vi "Main_System.back.vi"(7 "LabVIEW Web Service Request":refnum<class "Web Request.lvclass">) -> ()   [LabVIEW 2016]
uses:
  <vilib>/wsapi/Web Request.lvclass
  SubVIs/System_States.ctl
panel:
  in  "Tab Control":enum32{"Page 1", "Page 2"}(tab)
  out "error IO":errorcluster
  out "JSON string":string
  out "runtime":dbl=-1.0 format="%#_13g"
  out "Cluster":T1
  in  "Debug Provide Metadata":bool
  in  "Debug Provide Metadata (file)":bool
  out "Next State":T2
  out "Output/Debug":T3={"Test_File"="", "Error"="OK", "RF_Center_Freq"="0", "RF_Gain"="0", "Status"="Done"}
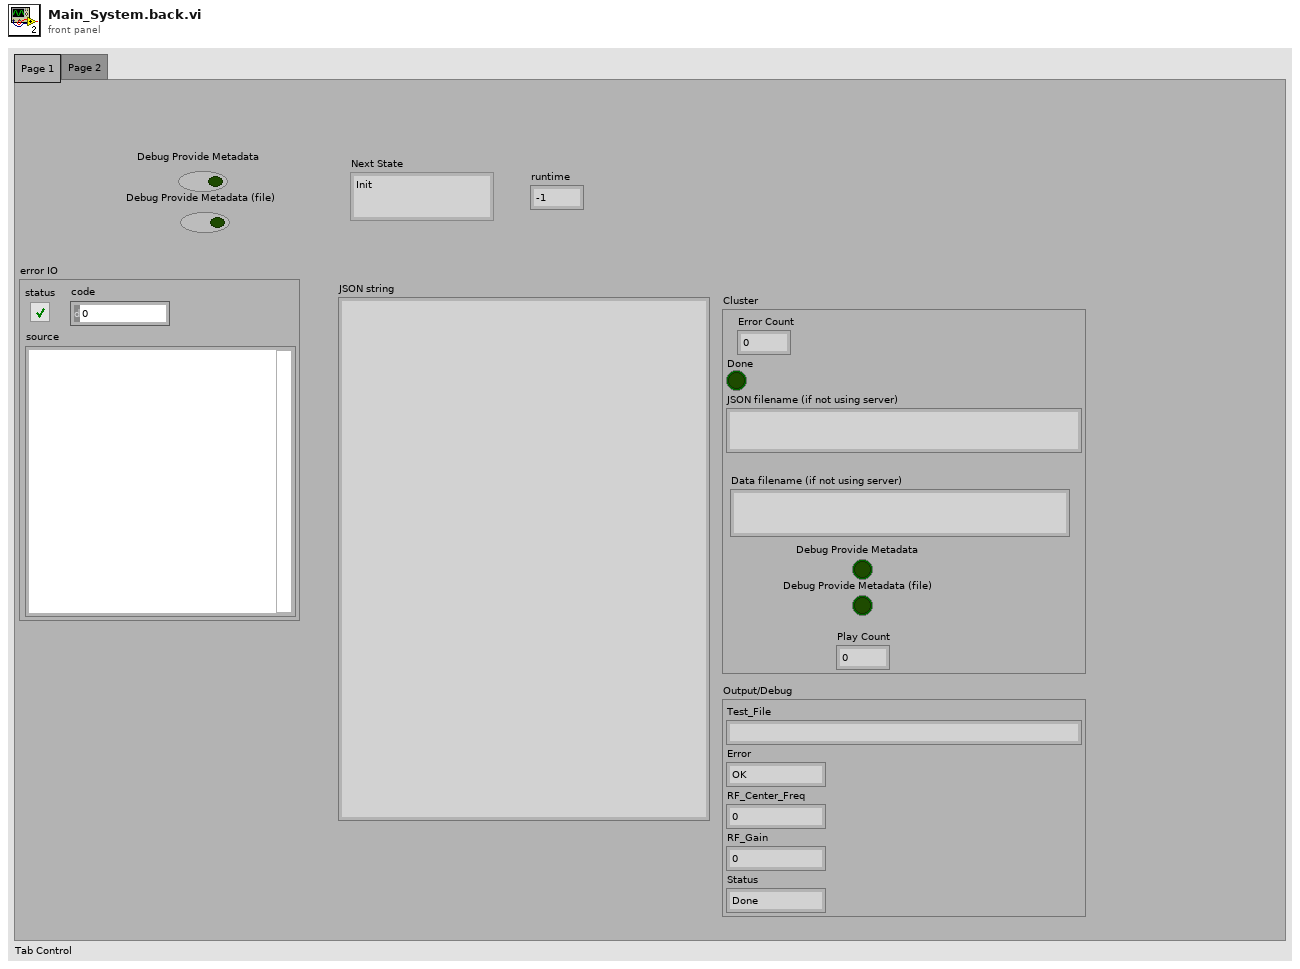
[diagram p1: front panel]
types:
  T1 = cluster{"Error Count":u64, "Done":bool, "JSON filename (if not using server)":string, "Data filename (if not using server)":string, "Debug Provide Metadata":bool, "Debug Provide Metadata (file)":bool, "Play Count":u64}
  T2 = typedef "System_States.ctl" = enum16{"Init", "Wait for Metadata", "Parse Metadata", "Play File", "Finished Playing", "Report Error", "Exit"}
  T3 = cluster{"Test_File":string, "Error":string, "RF_Center_Freq":string, "RF_Gain":string, "Status":string}
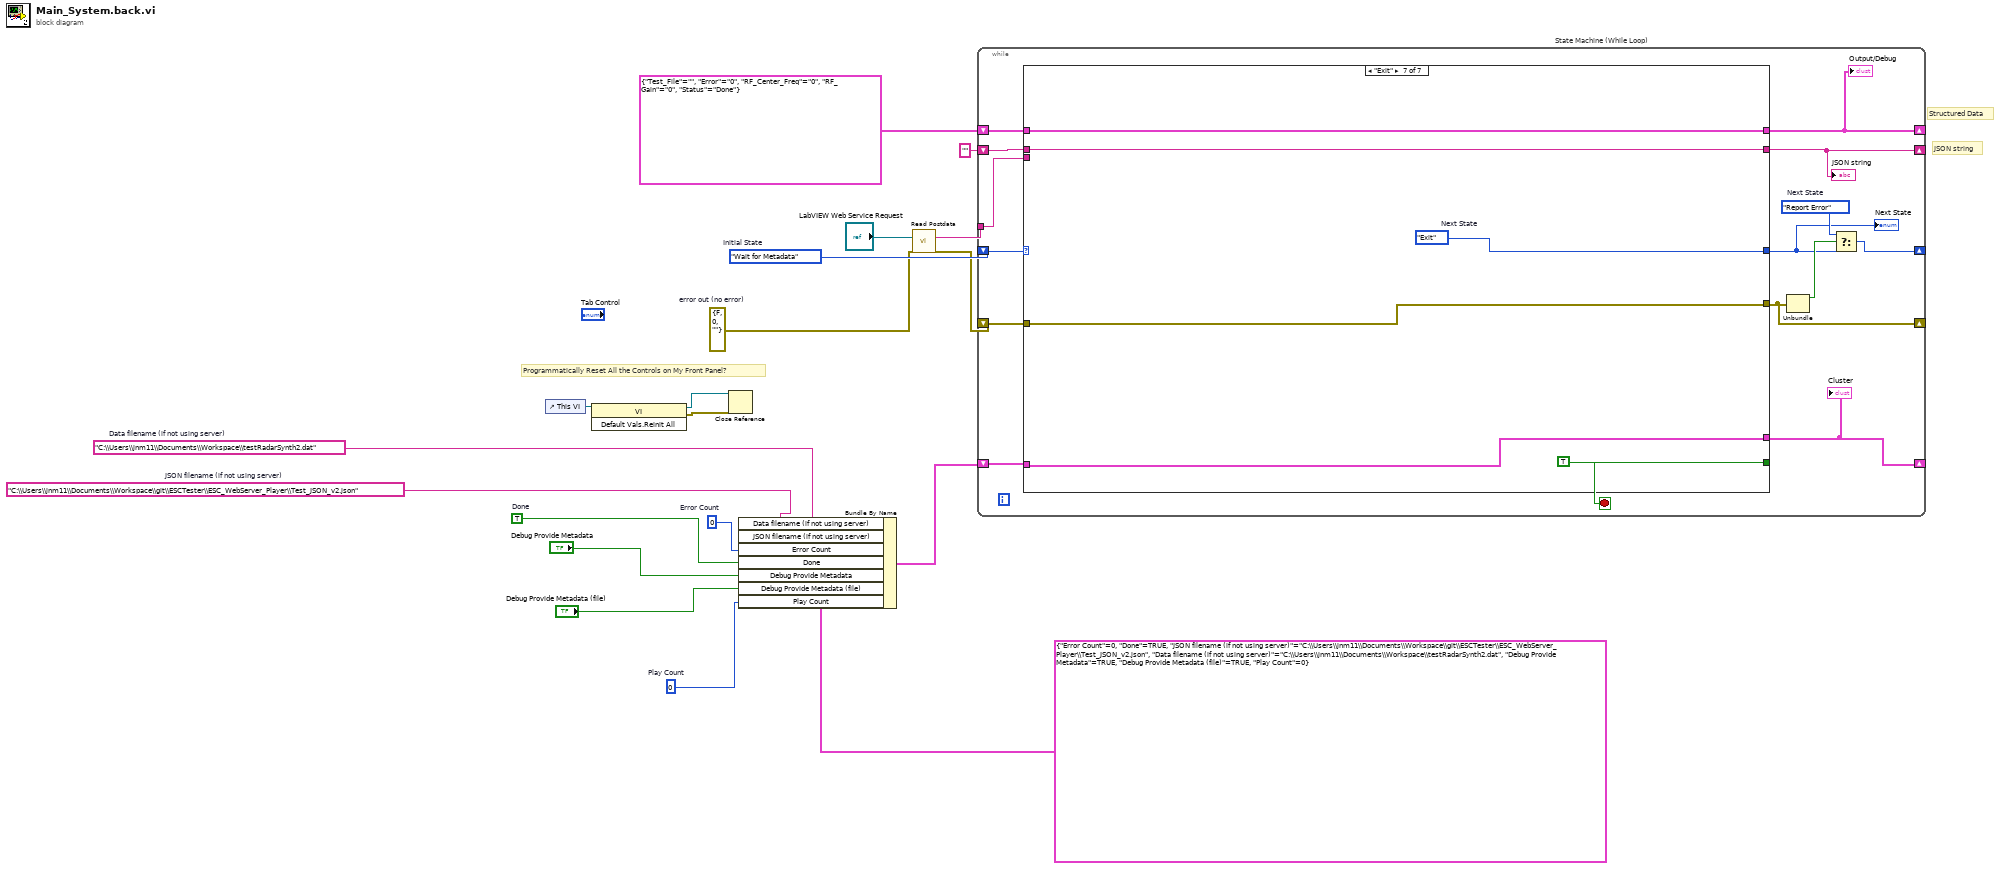
[diagram p0: block diagram]
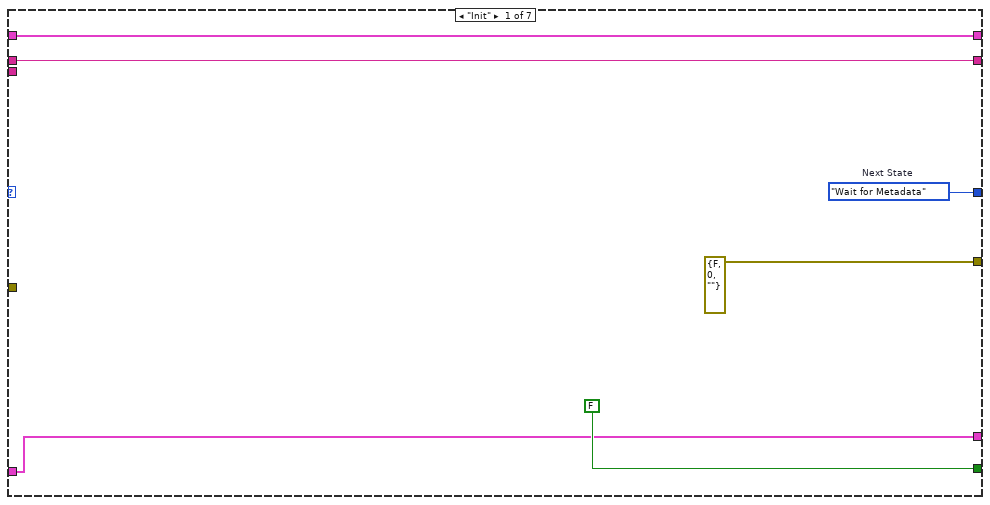
[diagram p2: hidden frame]
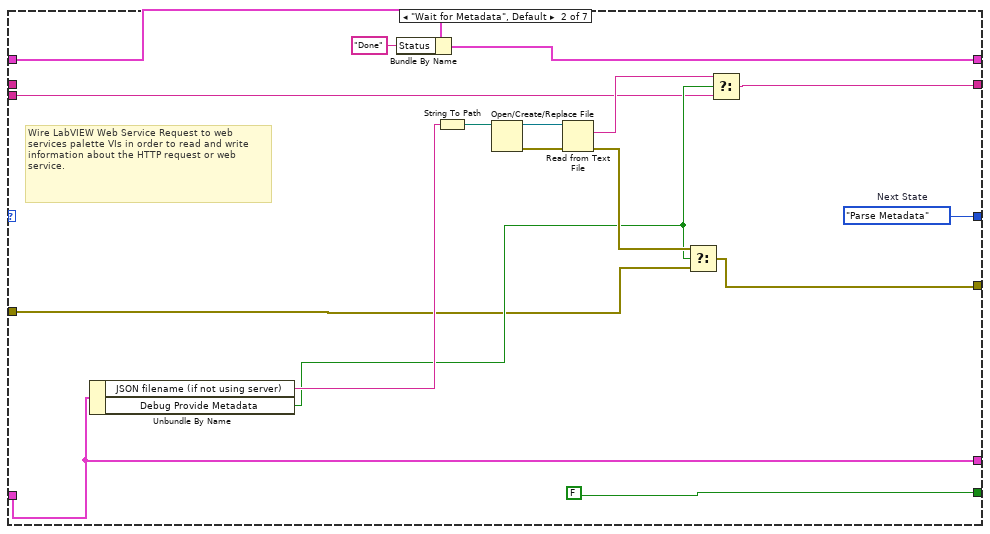
[diagram p3: hidden frame]
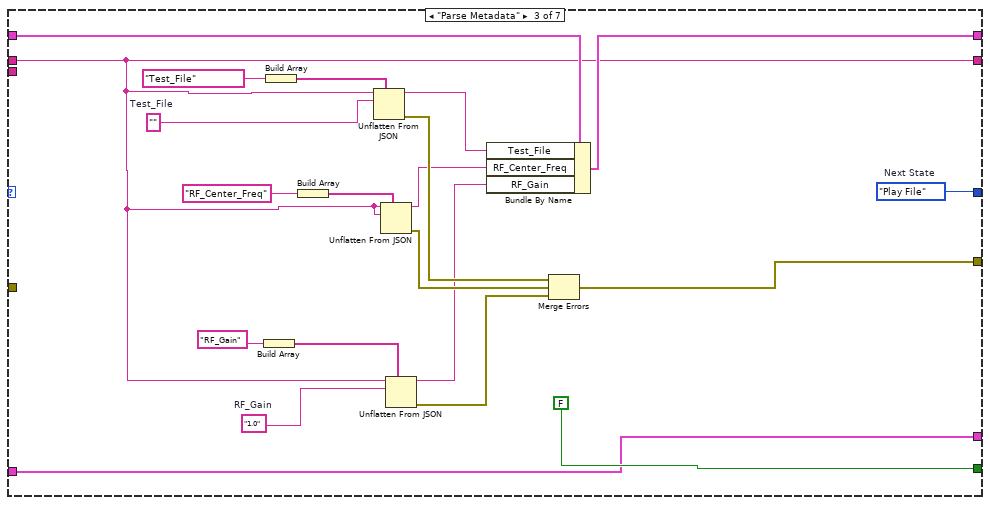
[diagram p4: hidden frame]
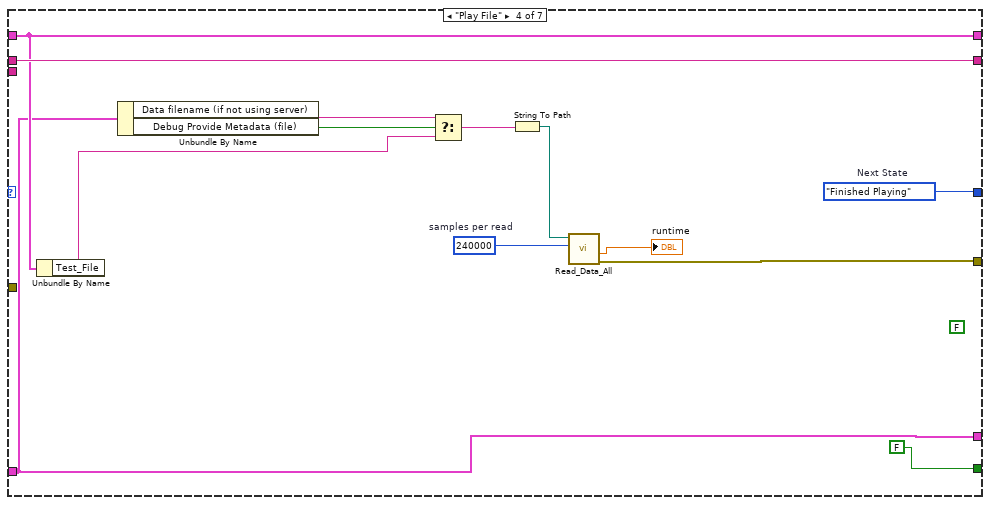
[diagram p5: hidden frame]
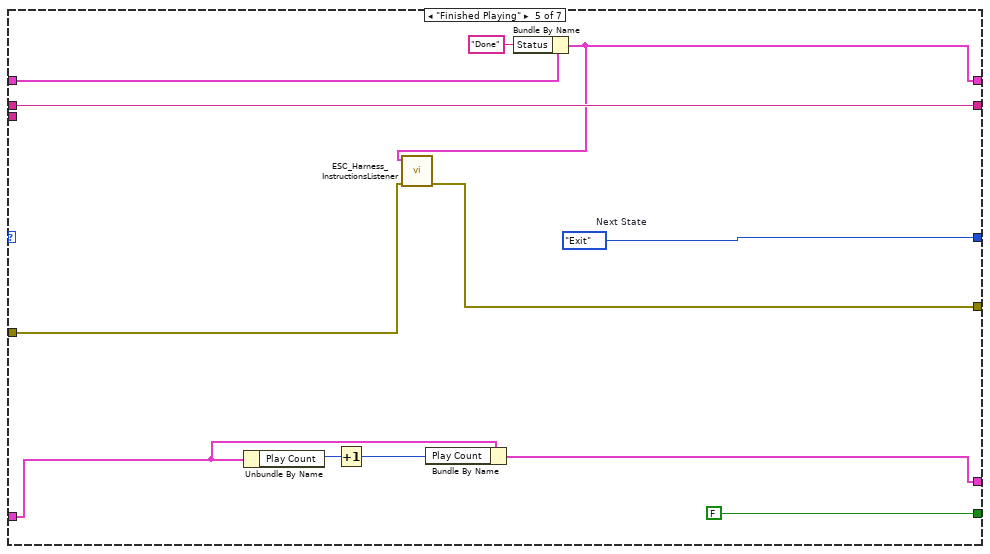
[diagram p6: hidden frame]
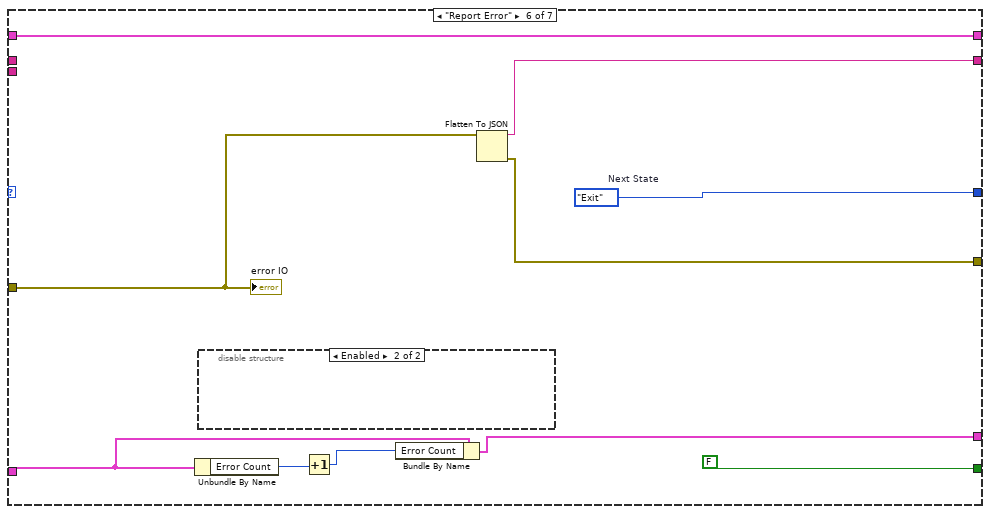
[diagram p7: hidden frame]
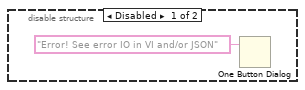
[diagram p8: hidden frame]
diagram:
  w9 = u64 0  # Play Count
  w15 = TRUE  # Done
  w16 = u64 0  # Error Count
  w10 = "C:\\Users\\jnm11\\Documents\\Workspace\\testRadarSynth2.dat"  # Data filename (if not using server)
  w17 = "C:\\Users\\jnm11\\Documents\\Workspace\\git\\ESCTester\\ESC_WebServer_Player\\Test_JSON_v2.json"  # JSON filename (if not using server)
  w7 = errorcluster {"status"=FALSE, "code"=0, "source"=""}  # error out (no error)
  w19 = System_States."Wait for Metadata"  # Initial State
  # "Programmatically Reset All the Controls on My Front Panel?"
  # "JSON string"
  # "Structured Data"
  n1 = control-ref of="This VI"() -> (w3:refnum<vi>)
  n2 = invoke class="VI" method="Default Vals.Reinit All"(reference=w3) -> (reference out=w2:refnum<vi>, error out=w1:errorcluster)  [unwired: 2 in, 1 out]
  n3 = Close Reference(reference=w2, error in (no error)=w1) -> ()  [unwired: 1 out]
  n4 = Bundle By Name(cluster=T1 {"Error Count"=0, "Done"=TRUE, "JSON filename (if not using server)"="C:\\Users\\jnm11\\Documents\\Workspace\\git\\ESCTester\\ESC_WebServer_Player\\Test_JSON_v2.json", "Data filename (if not using server)"="C:\\Users\\jnm11\\Documents\\Workspace\\testRadarSynth2.dat", "Debug Provide Metadata"=TRUE, "Debug Provide Metadata (file)"=TRUE, "Play Count"=0}, "Data filename (if not using server)"=w10, "JSON filename (if not using server)"=w17, "Error Count"=w16, "Done"=w15, "Debug Provide Metadata"="Debug Provide Metadata", "Debug Provide Metadata (file)"="Debug Provide Metadata (file)", "Play Count"=w9) -> (w12:T1)
  n5 = call <vilib>:"Read Postdata.vi"("LabVIEW Web Service Request"="LabVIEW Web Service Request", "error in (no error)"=w7) -> ("postdata"=w4:string, "error out"=w6:errorcluster)  [unwired: 11 in, 1 out]
  n6 = while "State Machine (While Loop)" {
    shift-right: [w30] -> _
    shift-left: w19 -> [w34]
    shift-right: [w26] -> _
    shift-left: "" ("JSON string") -> [w32]
    shift-right: [w20] -> _
    shift-left: T3 {"Test_File"="", "Error"="0", "RF_Center_Freq"="0", "RF_Gain"="0", "Status"="Done"} -> [w31]
    shift-right: [w29] -> _
    shift-left: w6 -> [w27]
    shift-right: [w24] -> _
    shift-left: w12 -> [w25]
    tunnel: w4 -> [w21]
    stop <- w33 stop-if-true
    w23 = System_States."Report Error"  # Next State
    n7 = case shown="\"Exit\"" w34 {
      tunnel: [FALSE FALSE FALSE FALSE FALSE FALSE TRUE] -> w33
      tunnel: [w39 w56 w67 w91 w102 w112 w119] -> w22
      tunnel: w32 -> [w37 _ w60 w90 w101 _ w118]
      tunnel: w31 -> [w38 w45 w71 w89 w94 w106 w117]
      tunnel: [w38 w44 w68 w89 w93 w106 w117] -> w20
      tunnel: [w37 w54 w60 w90 w101 w109 w118] -> w26
      tunnel: [errorcluster {"status"=FALSE, "code"=0, "source"=""} ("error IO") w55 w63 w79 w95 w111 w116] -> w29
      tunnel: w27 -> [_ w42 _ _ w96 w110 w116]
      tunnel: w25 -> [w35 w46 w61 w81 w98 w104 w115]
      tunnel: [w35 w46 w61 w81 w97 w105 w115] -> w24
      tunnel: w21 -> [_ w43 _ _ _ _ _]
      frame "Init" {
        w39 = System_States."Wait for Metadata"  # Next State
      }
      frame "Wait for Metadata", Default {
        w56 = System_States."Parse Metadata"  # Next State
        # "Wire LabVIEW Web Service Request to web services palette VIs in order to read and write information about the HTTP request or web service."
        n8 = Unbundle By Name(w46) -> ("JSON filename (if not using server)"=w48:string, "Debug Provide Metadata"=w47:bool)
        n9 = Bundle By Name(cluster=w45, "Status"="Done") -> (w44:T3)
        n10 = String To Path(string=w48) -> (path=w49:path)
        n11 = Open/Create/Replace File(file path (use dialog)=w49) -> (refnum out=w53:refnum<file>, error out=w52:errorcluster)  [unwired: 5 in, 1 out]
        n12 = Read from Text File(file (use dialog)=w53, error in=w52) -> (text=w50:string, error out=w51:errorcluster)  [unwired: 2 in, 2 out]
        n13 = Select(t=w51, s=w47, f=w42) -> (s? t:f=w55:errorcluster)
        n14 = Select(t=w50, s=w47, f=w43) -> (s? t:f=w54:string)
      }
      frame "Parse Metadata" {
        w62 = "1.0"  # RF_Gain
        w67 = System_States."Play File"  # Next State
        w69 = ""  # Test_File
        n15 = Build Array("RF_Gain") -> (w74:string[])
        n16 = Build Array("Test_File") -> (w72:string[])
        n17 = Build Array("RF_Center_Freq") -> (w73:string[])
        n18 = Unflatten From JSON(path=w72, JSON string=w60, type and defaults=w69) -> (value=w70:string, error out=w66:errorcluster)  [unwired: 4 in]
        n19 = Unflatten From JSON(path=w73, JSON string=w60, type and defaults=w60) -> (value=w59:string, error out=w65:errorcluster)  [unwired: 4 in]
        n20 = Unflatten From JSON(path=w74, JSON string=w60, type and defaults=w62) -> (value=w58:string, error out=w64:errorcluster)  [unwired: 4 in]
        n21 = Bundle By Name(cluster=w71, "Test_File"=w70, "RF_Center_Freq"=w59, "RF_Gain"=w58) -> (w68:T3)
        n22 = Merge Errors(w66, w65, w64) -> (w63:errorcluster)
      }
      frame "Play File" {
        w87 = 240000  # samples per read
        (unwired) FALSE ("is Done")
        w91 = System_States."Finished Playing"  # Next State
        n23 = Unbundle By Name(w89) -> ("Test_File"=w82:string)
        n24 = Unbundle By Name(w81) -> ("Data filename (if not using server)"=w85:string, "Debug Provide Metadata (file)"=w86:bool)
        n25 = Select(t=w85, s=w86, f=w82) -> (s? t:f=w84:string)
        n26 = String To Path(string=w84) -> (path=w83:path)
        n27 = call "Read_Data_All.vi"("samples per read"=w87, "path"=w83) -> ("error out"=w79:errorcluster, "runtime (ms)"=→"runtime":dbl)  [unwired: 6 in, 2 out]
      }
      frame "Finished Playing" {
        w102 = System_States."Exit"  # Next State
        n28 = Unbundle By Name(w98) -> ("Play Count"=w100:u64)
        n29 = Increment(x=w100) -> (x+1=w99:u64)
        n30 = Bundle By Name(cluster=w98, "Play Count"=w99) -> (w97:T1)
        n31 = Bundle By Name(cluster=w94, "Status"="Done") -> (w93:T3)
        n32 = call "ESC_Harness_InstructionsListener.vi"("error in (no error)"=w96, "Input"=w93) -> ("error out"=w95:errorcluster)  [unwired: 8 in]
      }
      frame "Report Error" {
        w112 = System_States."Exit"  # Next State
        n33 = Unbundle By Name(w104) -> ("Error Count"=w108:u64)
        n34 = disable-structure shown="Enabled" {
          frame Disabled {
            n35 = One Button Dialog(message="Error! See error IO in VI and/or JSON") -> ()  [unwired: 1 in, 1 out]
          }
          frame Enabled {
          }
        }
        n36 = Increment(x=w108) -> (x+1=w107:u64)
        n37 = Bundle By Name(cluster=w104, "Error Count"=w107) -> (w105:T1)
        n38 = Flatten To JSON(anything=w110) -> (JSON string=w109:string, 11:w111:errorcluster)  [unwired: 2 in]
        "error IO" <- w110
      }
      frame "Exit" {
        w119 = System_States."Exit"  # Next State
      }
    }
    "JSON string" <- w26
    "Cluster" <- w24
    "Next State" <- w22
    "Output/Debug" <- w20
    n39 = Unbundle(w29) -> ("status"=w28:bool)  [unwired: 2 out]
    n40 = Select(t=w23, s=w28, f=w22) -> (s? t:f=w30:T2)
  }
